vi "Retrieve_PackageImage.vi"(8 "error in (no error)":errorcluster, 10 "Image Filepath":path, 11 "AppImage Properties":T1) -> (0 "error out":errorcluster)   [LabVIEW 2021]
uses:
  TypeDefs/AppImageProperties.ctl
  TypeDefs/FPGA_Properties_Element.ctl
  <userlib>/_OpenG.lib/lvzip/lvzip.llb/ZLIB Open ZIP Mode__ogtk.ctl
  3bfd12fe-abaa-4926-9c30-3254df856dbe.vi
  <vilib>/JDP Science/JSONtext/Variant to JSON Text.vi
  <userlib>/_OpenG.lib/lvzip/lvzip.llb/subVI/ZLIB Open Zip Archive (Path)__ogtk.vi
  <userlib>/_OpenG.lib/lvzip/lvzip.llb/subVI/ZLIB Store File (Path)__ogtk.vi
  <vilib>/JDP Science/JSONtext/LVClass Serializer/JSONtext LVClass Serializer.lvclass
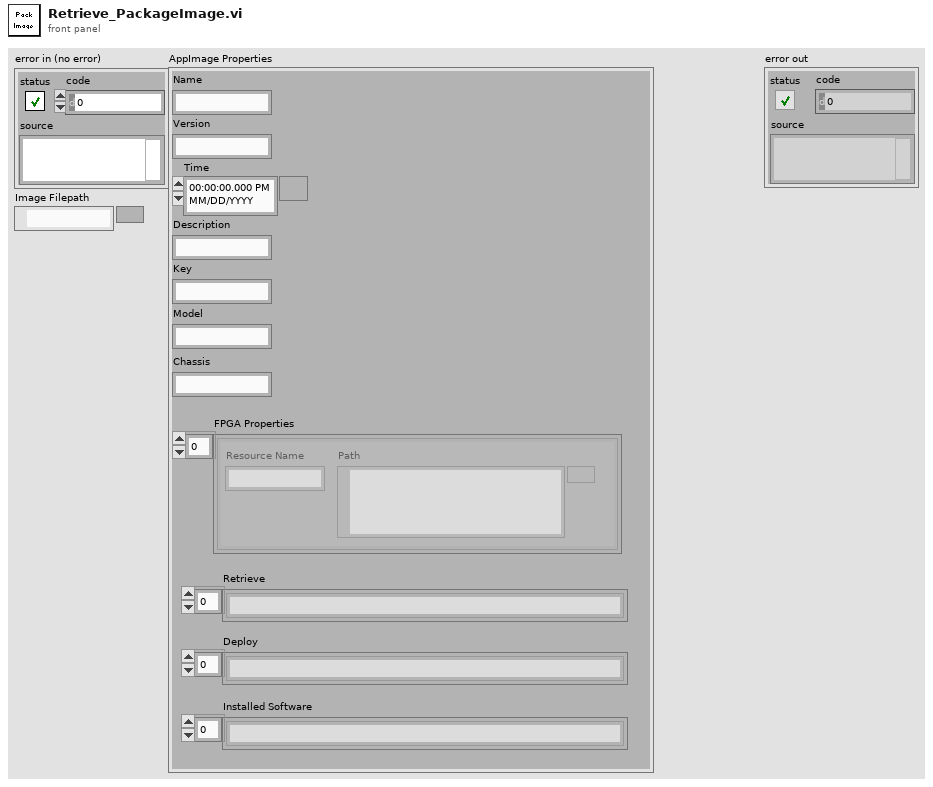
[diagram p1: front panel]
types:
  T1 = typedef "AppImageProperties.ctl" = cluster{"Name":string, "Version":string, "Time":timestamp, "Description":string, "Key":string, "Chassis":string, "FPGA Properties":T2[], "Model":string, "Retrieve":string[], "Deploy":string[], "Installed Software":string[]}
  T2 = typedef "FPGA_Properties_Element.ctl" = cluster{"Resource Name":string, "Path":path}
  T3 = typedef "ZLIB Open ZIP Mode__ogtk.ctl" = enum16{"create new", "append to end", "append to archive"}
  T4 = enum16{"open", "replace", "create", "open or create", "replace or create", "replace or create with confirmation"}
  T5 = typedef "ZLIB Zip Handle__ogtk.ctl" = refnum<k1>
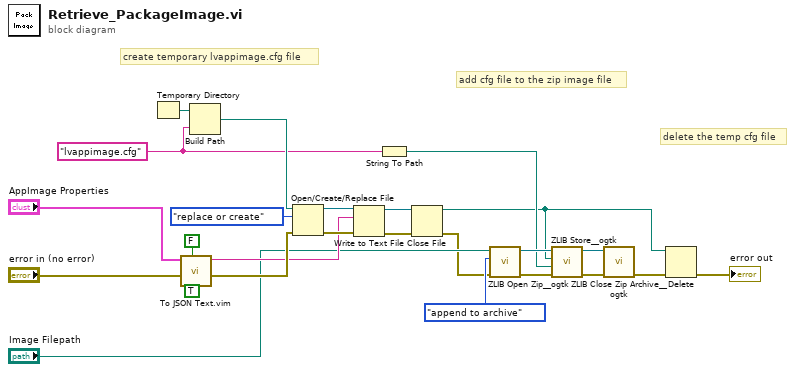
[diagram p0: block diagram]
diagram:
  w12 = "lvappimage.cfg"
  # "delete the temp cfg file"
  # "add cfg file to the zip image file"
  # "create temporary lvappimage.cfg file"
  n1 = Temporary Directory() -> (w21:path)
  n2 = call "To JSON Text.vim"("Pretty Print?"=TRUE, "enable LabVIEW extensions? (T)"=FALSE, "error in (no error)"="error in (no error)", "Anything"="AppImage Properties") -> ("error out"=w17:errorcluster, "<JSON>"=w15:string)  [unwired: 6 in]
  n3 = Build Path(base path=w21, name or relative path=w12) -> (appended path=w18:path)
  n4 = Open/Create/Replace File(file path (use dialog)=w18, error in=w17, operation (0:open)=T4."replace or create") -> (refnum out=w20:refnum<file>, error out=w16:errorcluster)  [unwired: 3 in, 1 out]
  n5 = Write to Text File(file (use dialog)=w20, text=w15, error in=w16) -> (refnum out=w14:refnum<file>, error out=w13:errorcluster)  [unwired: 1 in, 1 out]
  n6 = String To Path(string=w12) -> (path=w6:path)
  n7 = Close File(refnum=w14, error in=w13) -> (path=w3:path, error out=w1:errorcluster)
  n8 = call-poly <userlib>:"ZLIB Open Zip__ogtk.vi"("error in (no error)"=w1, "append (create new)"=ZLIB_Open_ZIP_Mode__ogtk."append to archive", "archive name"="Image Filepath") -> ("error out"=w4:errorcluster, "zip Refnum"=w9:T5)  [unwired: 2 in, 1 out]
  n9 = call-poly <userlib>:"ZLIB Store__ogtk.vi"("error in (no error)"=w4, "internal name (same as source name)"=w6, "source path"=w3, "zip Refnum"=w9) -> ("error out"=w5:errorcluster, "zip Refnum out"=w8:T5)  [unwired: 6 in]
  n10 = call <userlib>:"ZLIB Close Zip Archive__ogtk.vi"("error in (no error)"=w5, "zip Refnum"=w8) -> ("error out"=w2:errorcluster)  [unwired: 4 in, 1 out]
  n11 = Delete(path (use dialog)=w3, error in=w2) -> (error out=→"error out":errorcluster)  [unwired: 3 in, 2 out]
